vi "unix_time.get.vi"(10 "Time Stamp (empty: now)":timestamp format="%<%x %.3X>T") -> (1 "Nano Seconds":i64, 2 "Epoch Time (s)":i64)   [LabVIEW 2020, in "Nominal Client.lvclass"]
uses:
  Nominal Client.lvclass
  <vilib>/LabVIEW Open Source Project/Epoch Date & Time/epoch.UNIX/Epoch.UNIX.lvclass
  C:/Program Files/National Instruments/LabVIEW 2020/vi.lib/LabVIEW Open Source Project/Epoch Date & Time/epoch/Epoch.lvclass
  Nominal Client.lvclass/Nominal Client.ctl
  C:/Program Files/National Instruments/LabVIEW 2020/vi.lib/LabVIEW Open Source Project/Epoch Date & Time/epoch.UNIX/Epoch.UNIX.lvclass
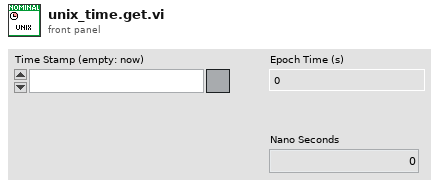
[diagram p1: front panel]
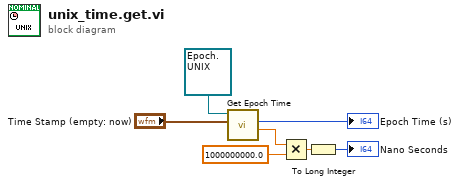
[diagram p0: block diagram]
diagram:
  n1 = call <vilib>:"Get Epoch Time.vi"("Timestamp (now)"="Time Stamp (empty: now)", "Epoch (Local)"=refnum<class "Epoch.UNIX.lvclass"> refnum ("Epoch.UNIX.lvclass")) -> ("Fractional Second"=w2:dbl, "Epoch Time (s)"=→"Epoch Time (s)":i64)  [unwired: 7 in, 1 out]
  n2 = Multiply(x=w2, y=1000000000.0) -> (x*y=w7:dbl)
  n3 = To Long Integer(number=w7) -> (32bit integer=→"Nano Seconds":i32)
